vi "Port table lookup.vi"(3 "error in (no error)":errorcluster, 5 "Port name":string) -> (0 "error out":errorcluster, 2 "Line":tag)   [LabVIEW 2015]
doc: "Searches the port table for the port name provided and returns the corresponding line"
uses:
  <vilib>/Utility/error.llb/DialogType.ctl
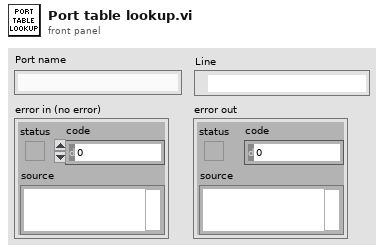
[diagram p1: front panel]
types:
  T1 = typedef "DialogType.ctl" = u16
  T2 = typedef "Port table entry.ctl" = cluster{"Name":string, "Line":tag}
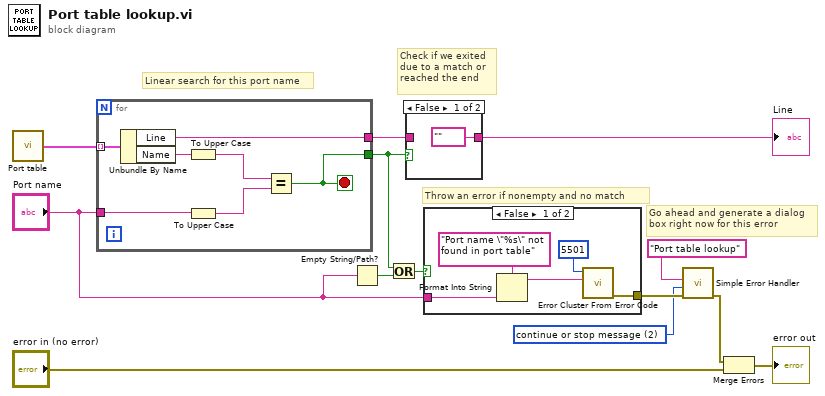
[diagram p0: block diagram]
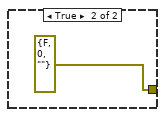
[diagram p2: hidden frame]
diagram:
  w2 = T1 2 items=["no dialog", "OK message", "continue or stop message", "OK message + warnings", "continue/stop + warnings"] ("type of dialog (OK msg:1)")
  # "Go ahead and generate a dialog\nbox right now for this error"
  # "Throw an error if nonempty and no match"
  # "Linear search for this port name"
  # "Check if we exited\ndue to a match or\nreached the end"
  n1 = call "Port table.vi"() -> ("Port table"=w13:T2[])
  n2 = for {
    tunnel: w13 -> [w20] mode=indexing
    tunnel: "Port name" -> [w17]
    tunnel: [w15] -> w12
    tunnel: [w14] -> w9
    stop <- w14 stop-if-true
    n3 = Unbundle By Name(w20) -> ("Line"=w15:tag, "Name"=w19:string)
    n4 = To Upper Case(1:w19) -> (0:w18:string)
    n5 = To Upper Case(1:w17) -> (0:w16:string)
    n6 = Equal?(x=w18, y=w16) -> (x = y?=w14:bool)
  }
  n7 = Empty String/Path?(string/path="Port name") -> (empty?=w10:bool)
  n8 = Or(x=w9, y=w10) -> (x .or. y?=w8:bool)
  n9 = case shown="False" w9 {
    tunnel: [tag "" ("Line") w22] -> w11
    tunnel: w12 -> [_ w22]
    frame False {
    }
    frame True {
    }
  }
  "Line" <- w11
  n10 = case shown="False" w8 {
    tunnel: "Port name" -> [w24 _]
    tunnel: [w23 errorcluster {"status"=FALSE, "code"=0, "source"=""} ("error out")] -> w4
    frame False {
      n11 = Format Into String(format string="Port name \"%s\" not found in port table", w24) -> (resulting string=w25:string)  [unwired: 2 in, 1 out]
      n12 = call <vilib>:"Error Cluster From Error Code.vi"("error message (\"\")"=w25, "error code (0)"=5501) -> ("error out"=w23:errorcluster)  [unwired: 7 in]
    }
    frame True {
    }
  }
  n13 = call <vilib>:"Simple Error Handler.vi"("error source (\" \")"="Port table lookup" ("error source (\" \")"), "type of dialog (OK msg:1)"=w2, "error in (no error)"=w4) -> ("error out"=w3:errorcluster)  [unwired: 2 in, 4 out]
  n14 = Merge Errors(w3, "error in (no error)") -> (→"error out":errorcluster)
